vi "Reset.vi"(8 "error in (no error)":errorcluster, 11 "HP3458aDMM in":refnum<class "HP3458aDMM.lvclass">) -> (0 "error out":errorcluster, 3 "HP3458aDMM out":refnum<class "HP3458aDMM.lvclass">)   [LabVIEW 2014, in "SamplerPlugins.lvlib" / "HP3458aDMM.lvclass"]
uses:
  HP3458aDMM.lvclass
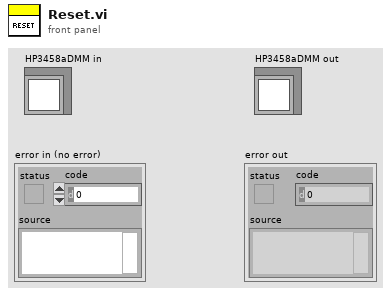
[diagram p1: front panel]
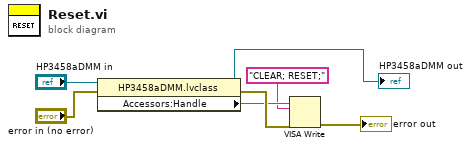
[diagram p0: block diagram]
diagram:
  n1 = property class="HP3458aDMM.lvclass"(reference="HP3458aDMM in", error in="error in (no error)") -> (reference out=→"HP3458aDMM out":refnum<class "HP3458aDMM.lvclass">, error out=w5:errorcluster, "Accessors:Handle"=w4:string)
  n2 = VISA Write(VISA resource name=w4, write buffer="CLEAR; RESET;", error in (no error)=w5) -> (error out=→"error out":errorcluster)  [unwired: 2 out]
